vi "Sensors Global Values.vi"() -> ()   [LabVIEW 2013]
panel:
  in  "Sensors Global Values":T1
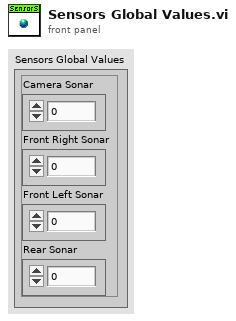
[diagram p1: front panel]
types:
  T1 = cluster{"Camera Sonar":dbl, "Front Right Sonar":dbl, "Front Left Sonar":dbl, "Rear Sonar":dbl}
diagram:
